vi "Autonomous Independent.vi"   [LabVIEW 2020]
doc: "This VI is called when autonomous begins, and will automatically be terminated when autonomous ends. You can carry out timed or sensor driven robot movement independently without needing to return to the caller."
uses:
  <vilib>/Rock Robotics/Network Tables/NT Read String.vi
  V1_nauru_2023_06_22/Global 1.vi
panel:
  # "Be sure to right-click and choose Data Operations>>Make Current Value default if you want to save the array values with the VI"
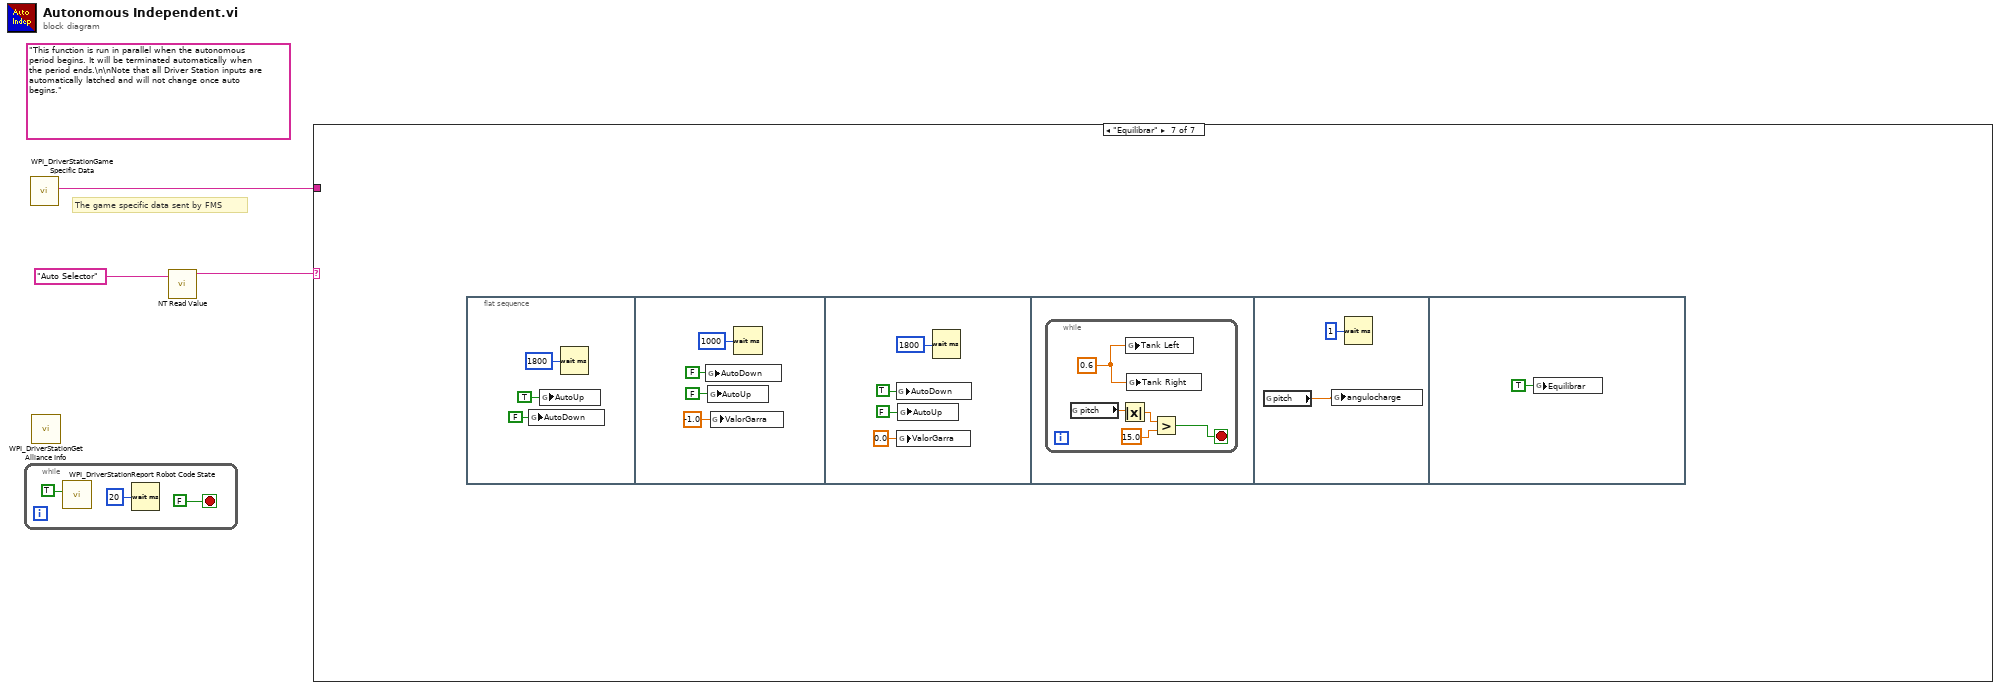
[diagram p0: block diagram]
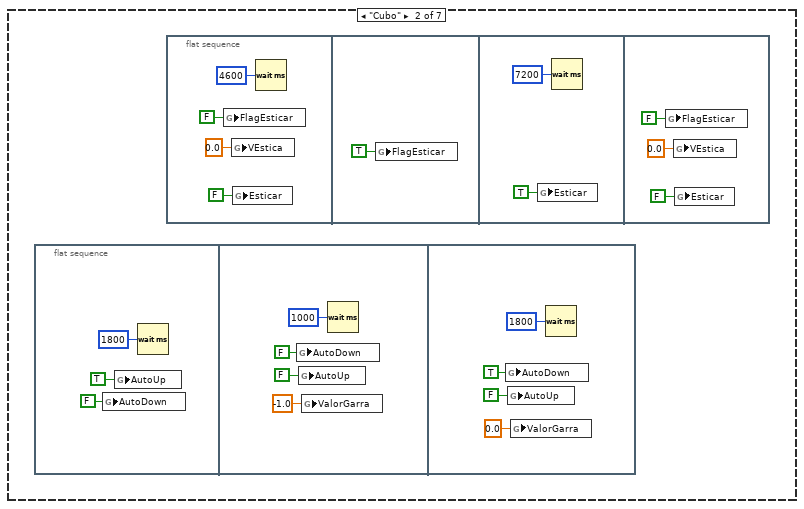
[diagram p3: hidden frame]
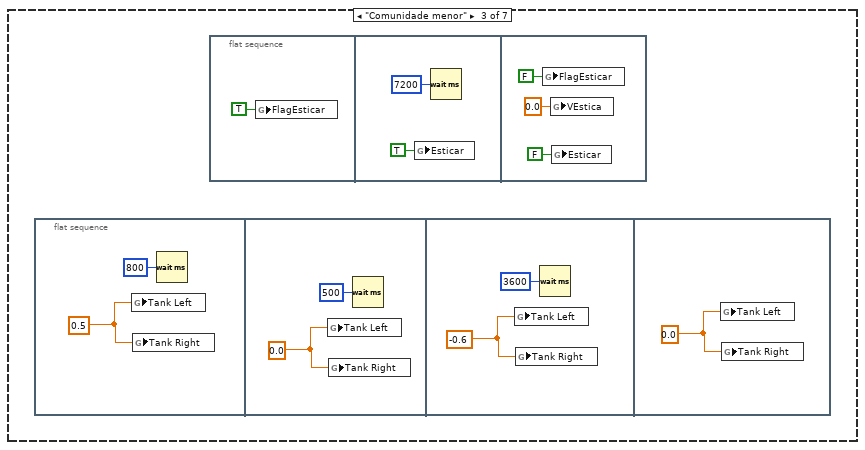
[diagram p4: hidden frame]
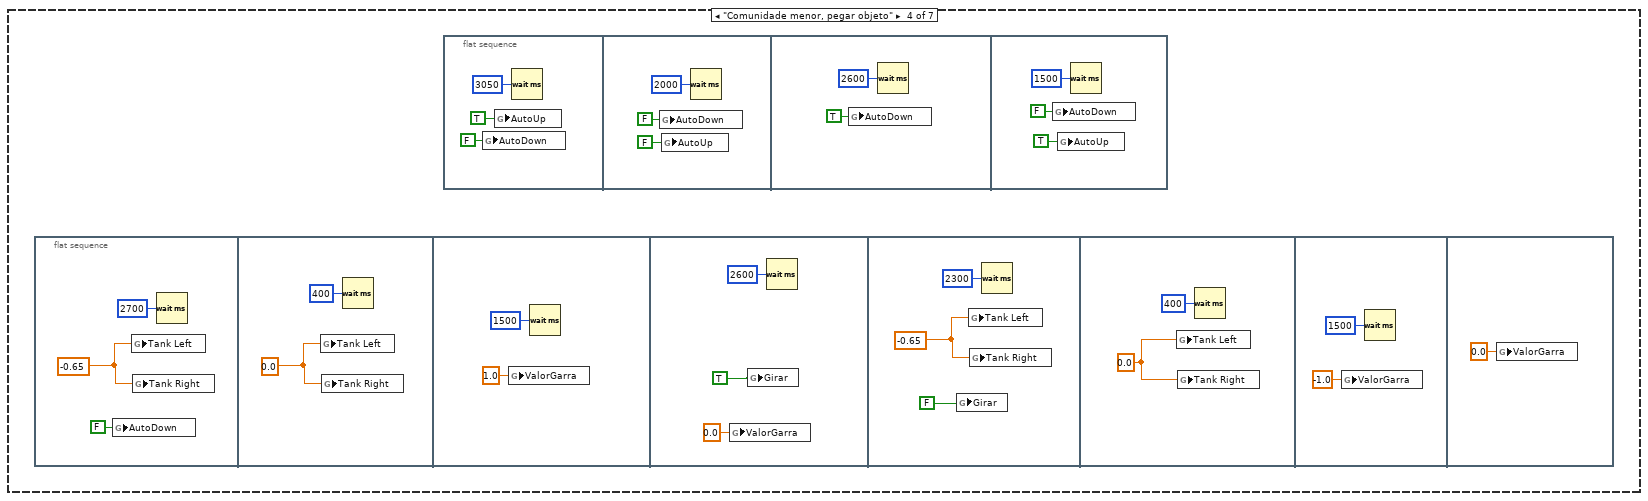
[diagram p5: hidden frame]
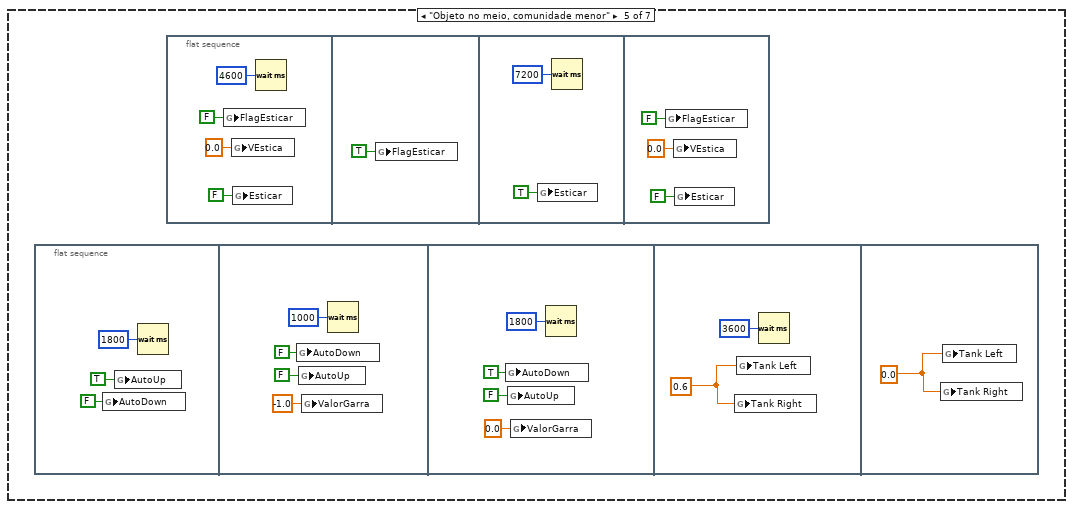
[diagram p6: hidden frame]
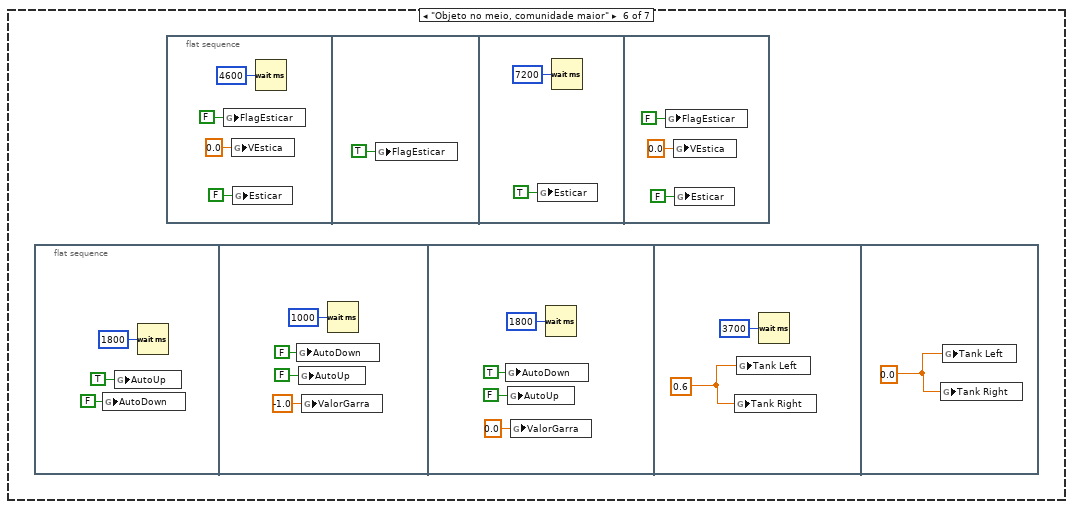
[diagram p7: hidden frame]
diagram:
  (unwired) "This function is run in parallel when the autonomous period begins. It will be terminated automatically when the period ends.\n\nNote that all Driver Station inputs are automatically latched and will not change once auto begins."
  # "The game specific data sent by FMS"
  n1 = while {
    stop <- FALSE stop-if-true
    n2 = call <vilib>:"WPI_DriverStationReport Robot Code State.vi"("Autonomous"=TRUE) -> ()  [unwired: 10 in, 1 out]
    n3 = Wait (ms)(milliseconds to wait=u32 20) -> ()  [unwired: 1 out]
  }
  n4 = call <vilib>:"WPI_DriverStationGame Specific Data.vi"() -> ("Game Specific Data"=w1:string)  [unwired: 11 in]
  n5 = call <vilib>:"WPI_DriverStationGet Alliance Info.vi"() -> ()  [unwired: 12 out]
  n6 = call-poly <vilib>:"NT Read Value.vi"("name"="Auto Selector" ("Name")) -> ("value"=w2:string)  [unwired: 8 in, 2 out]
  n7 = case shown="\"Equilibrar\"" w2 {
    tunnel: w1 -> [_ _ _ _ _ _ _]
    frame "Nada", Default {
    }
    frame "Cubo" {
      n8 = flat-sequence {
        frame #0 {
          n9 = global write "Global 1.vi" "AutoDown"(FALSE ("AutoUp")) -> ()
          n10 = global write "Global 1.vi" "AutoUp"(TRUE ("AutoUp")) -> ()
          n11 = Wait (ms)(milliseconds to wait=u32 1800) -> ()  [unwired: 1 out]
        }
        frame #1 {
          n12 = global write "Global 1.vi" "AutoDown"(FALSE ("AutoUp")) -> ()
          n13 = global write "Global 1.vi" "AutoUp"(FALSE ("AutoUp")) -> ()
          n14 = global write "Global 1.vi" "ValorGarra"(-1.0 ("ValorGarra")) -> ()
          n15 = Wait (ms)(milliseconds to wait=u32 1000) -> ()  [unwired: 1 out]
        }
        frame #2 {
          n16 = global write "Global 1.vi" "AutoDown"(TRUE ("AutoUp")) -> ()
          n17 = global write "Global 1.vi" "AutoUp"(FALSE ("AutoUp")) -> ()
          n18 = global write "Global 1.vi" "ValorGarra"(0.0 ("ValorGarra")) -> ()
          n19 = Wait (ms)(milliseconds to wait=u32 1800) -> ()  [unwired: 1 out]
        }
      }
      n20 = flat-sequence {
        frame #0 {
          n21 = global write "Global 1.vi" "FlagEsticar"(FALSE ("Retrair")) -> ()
          n22 = global write "Global 1.vi" "VEstica"(0.0 ("VEstica")) -> ()
          n23 = global write "Global 1.vi" "Esticar"(FALSE ("Retrair")) -> ()
          n24 = Wait (ms)(milliseconds to wait=u32 4600) -> ()  [unwired: 1 out]
        }
        frame #1 {
          n25 = global write "Global 1.vi" "FlagEsticar"(TRUE ("Retrair")) -> ()
        }
        frame #2 {
          n26 = global write "Global 1.vi" "Esticar"(TRUE ("Retrair")) -> ()
          n27 = Wait (ms)(milliseconds to wait=u32 7200) -> ()  [unwired: 1 out]
        }
        frame #3 {
          n28 = global write "Global 1.vi" "FlagEsticar"(FALSE ("Retrair")) -> ()
          n29 = global write "Global 1.vi" "VEstica"(0.0 ("VEstica")) -> ()
          n30 = global write "Global 1.vi" "Esticar"(FALSE ("Retrair")) -> ()
        }
      }
    }
    frame "Comunidade menor" {
      n31 = flat-sequence {
        frame #0 {
          w35 = 0.5 ("Tank Left")
          n32 = global write "Global 1.vi" "Tank Left"(w35) -> ()
          n33 = global write "Global 1.vi" "Tank Right"(w35) -> ()
          n34 = Wait (ms)(milliseconds to wait=u32 800) -> ()  [unwired: 1 out]
        }
        frame #1 {
          w37 = 0.0 ("Tank Left")
          n35 = global write "Global 1.vi" "Tank Left"(w37) -> ()
          n36 = global write "Global 1.vi" "Tank Right"(w37) -> ()
          n37 = Wait (ms)(milliseconds to wait=u32 500) -> ()  [unwired: 1 out]
        }
        frame #2 {
          w39 = -0.6 ("Tank Left")
          n38 = global write "Global 1.vi" "Tank Left"(w39) -> ()
          n39 = global write "Global 1.vi" "Tank Right"(w39) -> ()
          n40 = Wait (ms)(milliseconds to wait=u32 3600) -> ()  [unwired: 1 out]
        }
        frame #3 {
          w40 = 0.0 ("Tank Left")
          n41 = global write "Global 1.vi" "Tank Left"(w40) -> ()
          n42 = global write "Global 1.vi" "Tank Right"(w40) -> ()
        }
      }
      n43 = flat-sequence {
        frame #0 {
          n44 = global write "Global 1.vi" "FlagEsticar"(TRUE ("Retrair")) -> ()
        }
        frame #1 {
          n45 = global write "Global 1.vi" "Esticar"(TRUE ("Retrair")) -> ()
          n46 = Wait (ms)(milliseconds to wait=u32 7200) -> ()  [unwired: 1 out]
        }
        frame #2 {
          n47 = global write "Global 1.vi" "FlagEsticar"(FALSE ("Retrair")) -> ()
          n48 = global write "Global 1.vi" "VEstica"(0.0 ("VEstica")) -> ()
          n49 = global write "Global 1.vi" "Esticar"(FALSE ("Retrair")) -> ()
        }
      }
    }
    frame "Comunidade menor, pegar objeto" {
      n50 = flat-sequence {
        frame #0 {
          w54 = -0.65 ("Tank Left")
          n51 = global write "Global 1.vi" "AutoDown"(FALSE ("AutoUp")) -> ()
          n52 = global write "Global 1.vi" "Tank Left"(w54) -> ()
          n53 = global write "Global 1.vi" "Tank Right"(w54) -> ()
          n54 = Wait (ms)(milliseconds to wait=u32 2700) -> ()  [unwired: 1 out]
        }
        frame #1 {
          w56 = 0.0 ("Tank Left")
          n55 = global write "Global 1.vi" "Tank Left"(w56) -> ()
          n56 = global write "Global 1.vi" "Tank Right"(w56) -> ()
          n57 = Wait (ms)(milliseconds to wait=u32 400) -> ()  [unwired: 1 out]
        }
        frame #2 {
          n58 = global write "Global 1.vi" "ValorGarra"(1.0 ("ValorGarra")) -> ()
          n59 = Wait (ms)(milliseconds to wait=u32 1500) -> ()  [unwired: 1 out]
        }
        frame #3 {
          n60 = global write "Global 1.vi" "ValorGarra"(0.0 ("ValorGarra")) -> ()
          n61 = global write "Global 1.vi" "Girar"(TRUE ("girar")) -> ()
          n62 = Wait (ms)(milliseconds to wait=u32 2600) -> ()  [unwired: 1 out]
        }
        frame #4 {
          w64 = -0.65 ("Tank Left")
          n63 = global write "Global 1.vi" "Girar"(FALSE ("girar")) -> ()
          n64 = global write "Global 1.vi" "Tank Left"(w64) -> ()
          n65 = global write "Global 1.vi" "Tank Right"(w64) -> ()
          n66 = Wait (ms)(milliseconds to wait=u32 2300) -> ()  [unwired: 1 out]
        }
        frame #5 {
          w65 = 0.0 ("Tank Left")
          n67 = global write "Global 1.vi" "Tank Left"(w65) -> ()
          n68 = global write "Global 1.vi" "Tank Right"(w65) -> ()
          n69 = Wait (ms)(milliseconds to wait=u32 400) -> ()  [unwired: 1 out]
        }
        frame #6 {
          n70 = global write "Global 1.vi" "ValorGarra"(-1.0 ("ValorGarra")) -> ()
          n71 = Wait (ms)(milliseconds to wait=u32 1500) -> ()  [unwired: 1 out]
        }
        frame #7 {
          n72 = global write "Global 1.vi" "ValorGarra"(0.0 ("ValorGarra")) -> ()
        }
      }
      n73 = flat-sequence {
        frame #0 {
          n74 = global write "Global 1.vi" "AutoDown"(FALSE ("AutoUp")) -> ()
          n75 = global write "Global 1.vi" "AutoUp"(TRUE ("AutoUp")) -> ()
          n76 = Wait (ms)(milliseconds to wait=u32 3050) -> ()  [unwired: 1 out]
        }
        frame #1 {
          n77 = global write "Global 1.vi" "AutoDown"(FALSE ("AutoUp")) -> ()
          n78 = global write "Global 1.vi" "AutoUp"(FALSE ("AutoUp")) -> ()
          n79 = Wait (ms)(milliseconds to wait=u32 2000) -> ()  [unwired: 1 out]
        }
        frame #2 {
          n80 = global write "Global 1.vi" "AutoDown"(TRUE ("AutoUp")) -> ()
          n81 = Wait (ms)(milliseconds to wait=u32 2600) -> ()  [unwired: 1 out]
        }
        frame #3 {
          n82 = global write "Global 1.vi" "AutoDown"(FALSE ("AutoUp")) -> ()
          n83 = global write "Global 1.vi" "AutoUp"(TRUE ("AutoUp")) -> ()
          n84 = Wait (ms)(milliseconds to wait=u32 1500) -> ()  [unwired: 1 out]
        }
      }
    }
    frame "Objeto no meio, comunidade menor" {
      n85 = flat-sequence {
        frame #0 {
          n86 = global write "Global 1.vi" "AutoDown"(FALSE ("AutoUp")) -> ()
          n87 = global write "Global 1.vi" "AutoUp"(TRUE ("AutoUp")) -> ()
          n88 = Wait (ms)(milliseconds to wait=u32 1800) -> ()  [unwired: 1 out]
        }
        frame #1 {
          n89 = global write "Global 1.vi" "AutoDown"(FALSE ("AutoUp")) -> ()
          n90 = global write "Global 1.vi" "AutoUp"(FALSE ("AutoUp")) -> ()
          n91 = global write "Global 1.vi" "ValorGarra"(-1.0 ("ValorGarra")) -> ()
          n92 = Wait (ms)(milliseconds to wait=u32 1000) -> ()  [unwired: 1 out]
        }
        frame #2 {
          n93 = global write "Global 1.vi" "AutoDown"(TRUE ("AutoUp")) -> ()
          n94 = global write "Global 1.vi" "AutoUp"(FALSE ("AutoUp")) -> ()
          n95 = global write "Global 1.vi" "ValorGarra"(0.0 ("ValorGarra")) -> ()
          n96 = Wait (ms)(milliseconds to wait=u32 1800) -> ()  [unwired: 1 out]
        }
        frame #3 {
          w92 = 0.6 ("Tank Left")
          n97 = global write "Global 1.vi" "Tank Right"(w92) -> ()
          n98 = global write "Global 1.vi" "Tank Left"(w92) -> ()
          n99 = Wait (ms)(milliseconds to wait=u32 3600) -> ()  [unwired: 1 out]
        }
        frame #4 {
          w93 = 0.0 ("Tank Left")
          n100 = global write "Global 1.vi" "Tank Right"(w93) -> ()
          n101 = global write "Global 1.vi" "Tank Left"(w93) -> ()
        }
      }
      n102 = flat-sequence {
        frame #0 {
          n103 = global write "Global 1.vi" "FlagEsticar"(FALSE ("Retrair")) -> ()
          n104 = global write "Global 1.vi" "VEstica"(0.0 ("VEstica")) -> ()
          n105 = global write "Global 1.vi" "Esticar"(FALSE ("Retrair")) -> ()
          n106 = Wait (ms)(milliseconds to wait=u32 4600) -> ()  [unwired: 1 out]
        }
        frame #1 {
          n107 = global write "Global 1.vi" "FlagEsticar"(TRUE ("Retrair")) -> ()
        }
        frame #2 {
          n108 = global write "Global 1.vi" "Esticar"(TRUE ("Retrair")) -> ()
          n109 = Wait (ms)(milliseconds to wait=u32 7200) -> ()  [unwired: 1 out]
        }
        frame #3 {
          n110 = global write "Global 1.vi" "FlagEsticar"(FALSE ("Retrair")) -> ()
          n111 = global write "Global 1.vi" "VEstica"(0.0 ("VEstica")) -> ()
          n112 = global write "Global 1.vi" "Esticar"(FALSE ("Retrair")) -> ()
        }
      }
    }
    frame "Objeto no meio, comunidade maior" {
      n113 = flat-sequence {
        frame #0 {
          n114 = global write "Global 1.vi" "AutoDown"(FALSE ("AutoUp")) -> ()
          n115 = global write "Global 1.vi" "AutoUp"(TRUE ("AutoUp")) -> ()
          n116 = Wait (ms)(milliseconds to wait=u32 1800) -> ()  [unwired: 1 out]
        }
        frame #1 {
          n117 = global write "Global 1.vi" "AutoDown"(FALSE ("AutoUp")) -> ()
          n118 = global write "Global 1.vi" "AutoUp"(FALSE ("AutoUp")) -> ()
          n119 = global write "Global 1.vi" "ValorGarra"(-1.0 ("ValorGarra")) -> ()
          n120 = Wait (ms)(milliseconds to wait=u32 1000) -> ()  [unwired: 1 out]
        }
        frame #2 {
          n121 = global write "Global 1.vi" "AutoDown"(TRUE ("AutoUp")) -> ()
          n122 = global write "Global 1.vi" "AutoUp"(FALSE ("AutoUp")) -> ()
          n123 = global write "Global 1.vi" "ValorGarra"(0.0 ("ValorGarra")) -> ()
          n124 = Wait (ms)(milliseconds to wait=u32 1800) -> ()  [unwired: 1 out]
        }
        frame #3 {
          w116 = 0.6 ("Tank Left")
          n125 = global write "Global 1.vi" "Tank Right"(w116) -> ()
          n126 = global write "Global 1.vi" "Tank Left"(w116) -> ()
          n127 = Wait (ms)(milliseconds to wait=u32 3700) -> ()  [unwired: 1 out]
        }
        frame #4 {
          w117 = 0.0 ("Tank Left")
          n128 = global write "Global 1.vi" "Tank Right"(w117) -> ()
          n129 = global write "Global 1.vi" "Tank Left"(w117) -> ()
        }
      }
      n130 = flat-sequence {
        frame #0 {
          n131 = global write "Global 1.vi" "FlagEsticar"(FALSE ("Retrair")) -> ()
          n132 = global write "Global 1.vi" "VEstica"(0.0 ("VEstica")) -> ()
          n133 = global write "Global 1.vi" "Esticar"(FALSE ("Retrair")) -> ()
          n134 = Wait (ms)(milliseconds to wait=u32 4600) -> ()  [unwired: 1 out]
        }
        frame #1 {
          n135 = global write "Global 1.vi" "FlagEsticar"(TRUE ("Retrair")) -> ()
        }
        frame #2 {
          n136 = global write "Global 1.vi" "Esticar"(TRUE ("Retrair")) -> ()
          n137 = Wait (ms)(milliseconds to wait=u32 7200) -> ()  [unwired: 1 out]
        }
        frame #3 {
          n138 = global write "Global 1.vi" "FlagEsticar"(FALSE ("Retrair")) -> ()
          n139 = global write "Global 1.vi" "VEstica"(0.0 ("VEstica")) -> ()
          n140 = global write "Global 1.vi" "Esticar"(FALSE ("Retrair")) -> ()
        }
      }
    }
    frame "Equilibrar" {
      n141 = flat-sequence {
        frame #0 {
          n142 = global write "Global 1.vi" "AutoDown"(FALSE ("AutoUp")) -> ()
          n143 = global write "Global 1.vi" "AutoUp"(TRUE ("AutoUp")) -> ()
          n144 = Wait (ms)(milliseconds to wait=u32 1800) -> ()  [unwired: 1 out]
        }
        frame #1 {
          n145 = global write "Global 1.vi" "AutoDown"(FALSE ("AutoUp")) -> ()
          n146 = global write "Global 1.vi" "AutoUp"(FALSE ("AutoUp")) -> ()
          n147 = global write "Global 1.vi" "ValorGarra"(-1.0 ("ValorGarra")) -> ()
          n148 = Wait (ms)(milliseconds to wait=u32 1000) -> ()  [unwired: 1 out]
        }
        frame #2 {
          n149 = global write "Global 1.vi" "AutoDown"(TRUE ("AutoUp")) -> ()
          n150 = global write "Global 1.vi" "ValorGarra"(0.0 ("ValorGarra")) -> ()
          n151 = global write "Global 1.vi" "AutoUp"(FALSE ("AutoUp")) -> ()
          n152 = Wait (ms)(milliseconds to wait=u32 1800) -> ()  [unwired: 1 out]
        }
        frame #3 {
          n153 = while {
            stop <- w129 stop-if-true
            w133 = 0.6 ("Tank Left")
            n154 = global read "Global 1.vi" "pitch"() -> (w132:dbl)
            n155 = Absolute Value(x=w132) -> (abs(x)=w131:dbl)
            n156 = global write "Global 1.vi" "Tank Left"(w133) -> ()
            n157 = global write "Global 1.vi" "Tank Right"(w133) -> ()
            n158 = Greater?(x=w131, y=15.0) -> (0:w129:bool)
          }
        }
        frame #4 {
          n159 = global read "Global 1.vi" "pitch"() -> (w134:dbl)
          n160 = global write "Global 1.vi" "angulocharge"(w134) -> ()
          n161 = Wait (ms)(milliseconds to wait=u32 1) -> ()  [unwired: 1 out]
        }
        frame #5 {
          n162 = global write "Global 1.vi" "Equilibrar"(TRUE ("Equilibrar")) -> ()
        }
      }
    }
  }
